vi "Read.vi"   [LabVIEW 2016, in "CVT.lvlib" / "Current Value Table.lvlib"]
doc: "This VI will read the data associated with a single tag. This VI will always look up the tag index if the name changes, or if index lookup failed previously (resulting in an error). This combines the functionality of the CVT2 VIs for reads and static reads."
uses:
  <vilib>/NI/Current Value Table/Current Value Table.lvlib
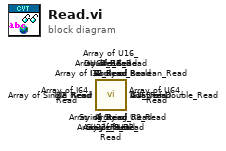
[diagram p0: block diagram]
diagram:
  n1 = call <vilib>:"Array of String_Read.vi"() -> ()  [unwired: 10 in, 2 out]
  n2 = call <vilib>:"Array of Boolean_Read.vi"() -> ()  [unwired: 10 in, 2 out]
  n3 = call <vilib>:"Array of Single_Read.vi"() -> ()  [unwired: 10 in, 2 out]
  n4 = call <vilib>:"Array of Double_Read.vi"() -> ()  [unwired: 10 in, 2 out]
  n5 = call <vilib>:"Array of I8_Read.vi"() -> ()  [unwired: 10 in, 2 out]
  n6 = call <vilib>:"Array of I16_Read.vi"() -> ()  [unwired: 10 in, 2 out]
  n7 = call <vilib>:"Array of I32_Read.vi"() -> ()  [unwired: 10 in, 2 out]
  n8 = call <vilib>:"Array of I64_Read.vi"() -> ()  [unwired: 10 in, 2 out]
  n9 = call <vilib>:"Array of U64_Read.vi"() -> ()  [unwired: 10 in, 2 out]
  n10 = call <vilib>:"Array of U32_Read.vi"() -> ()  [unwired: 10 in, 2 out]
  n11 = call <vilib>:"Array of U16_Read.vi"() -> ()  [unwired: 10 in, 2 out]
  n12 = call <vilib>:"Array of U8_Read.vi"() -> ()  [unwired: 10 in, 2 out]
  n13 = call <vilib>:"Boolean_Read.vi"() -> ()  [unwired: 10 in, 2 out]
  n14 = call <vilib>:"String_Read.vi"() -> ()  [unwired: 10 in, 2 out]
  n15 = call <vilib>:"U8_Read.vi"() -> ()  [unwired: 10 in, 2 out]
  n16 = call <vilib>:"U16_Read.vi"() -> ()  [unwired: 10 in, 2 out]
  n17 = call <vilib>:"U32_Read.vi"() -> ()  [unwired: 10 in, 2 out]
  n18 = call <vilib>:"U64_Read.vi"() -> ()  [unwired: 10 in, 2 out]
  n19 = call <vilib>:"I8_Read.vi"() -> ()  [unwired: 10 in, 2 out]
  n20 = call <vilib>:"I16_Read.vi"() -> ()  [unwired: 10 in, 2 out]
  n21 = call <vilib>:"I32_Read.vi"() -> ()  [unwired: 10 in, 2 out]
  n22 = call <vilib>:"I64_Read.vi"() -> ()  [unwired: 10 in, 2 out]
  n23 = call <vilib>:"Single_Read.vi"() -> ()  [unwired: 10 in, 2 out]
  n24 = call <vilib>:"Double_Read.vi"() -> ()  [unwired: 10 in, 2 out]
